vi "Test Broadcast Unfiltered Debug Log Not Filtered by Message.vi"(8 "error in (no error)":errorcluster, 11 "Test Case In":refnum<class "Debugger Test.lvclass">) -> (0 "error out":errorcluster, 3 "Test Case Out":refnum<class "Debugger Test.lvclass">)   [LabVIEW 2020, in "Debugger Test.lvclass"]
uses:
  Debugger Test.lvclass
  C:/Program Files (x86)/National Instruments/LabVIEW 2020/vi.lib/Astemes/LUnit/Test Case.lvclass
  source/Debugger/Debugger.lvclass
  C:/Users/anton/Documents/GitHub/triarc-debugger/source/Process/Debug Process.lvclass
  source/Debug Data/Raw Debug Data.ctl
  source/Debug Data/Debug Data.lvclass/Debug Data.ctl
  source/Process/Debug Process.lvclass/Debug Process.ctl
  <vilib>/Astemes/LUnit/Test Case.lvclass/Test Case.ctl
  <vilib>/Astemes/LUnit/LUnit Assertion Result.lvclass/LUnit Assertion Result.ctl
  <vilib>/Astemes/LUnit/LUnit Test Case Result.lvclass/LUnit Test Case Result.ctl
  <vilib>/Astemes/LUnit/LUnit Method Result.lvclass/LUnit Method Result.ctl
  01074fa8-ee8a-411d-bc8b-fc92c4f90959.vi
  source/Process/Public/Lifecycle/Get Lifecycle State.vi
  source/Process/Private/SubVIs/Wait for finish.vi
  source/Process/Protected/Messaging/Enqueue Message.vi
  source/Process/Private/SubVIs/Set Lifecycle State.vi
  <vilib>/Astemes/LUnit/Palette/Pass.vi
  <vilib>/Astemes/LUnit/Palette/Fail.vi
  <vilib>/Astemes/LUnit/Compare Variants.vi
  <vilib>/Astemes/LUnit/Describe Comparison.vi
  <vilib>/Astemes/LUnit/Set Assertion Type.vi
  <vilib>/Utility/error.llb/Clear Errors.vi
  <vilib>/Astemes/LUnit/Add test result.vi
  <vilib>/Astemes/LUnit/LUnit Write Passed.vi
  <vilib>/Astemes/LUnit/LUnit Write Message.vi
  <vilib>/Astemes/LUnit/LUnit Write Description.vi
  <vilib>/Astemes/LUnit/Variant to string.vi
  <vilib>/Astemes/LUnit/LUnit Write Assertion Type.vi
  <vilib>/Astemes/LUnit/LUnit Record Assertion Result.vi
  <vilib>/Astemes/LUnit/LUnit Aggregate Assertion Results.vi
  <vilib>/Astemes/LUnit/Assertion Result/LUnit Read Status.vi
  <vilib>/Astemes/LUnit/LUnit Read Message.vi
  <vilib>/Astemes/LUnit/LUnit Read Description.vi
  <vilib>/Astemes/LUnit/Method Result/LUnit Merge Status.vi
  <vilib>/Astemes/LUnit/LUnit Concatenate result strings.vi
  <vilib>/Utility/error.llb/Error Cluster From Error Code.vi
  <vilib>/Utility/Data Type/Get Type Information.vi
  <vilib>/Utility/LVClass/Get LV Class Name.vi
  <vilib>/Astemes/LUnit/LUnit Assertion Result.lvclass
  source/Process/Debug Process.lvclass
  source/Debug Data/Debug Data.lvclass
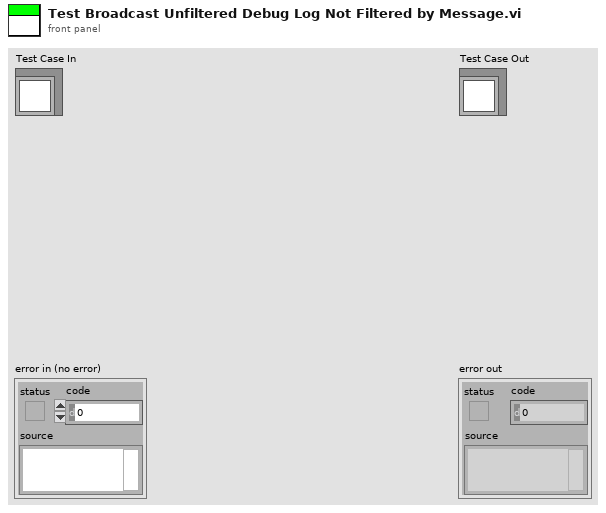
[diagram p1: front panel]
types:
  T1 = typedef "Debug Data.lvclass/Raw Debug Data.ctl" = cluster{"Action":string, "Call Chain":string, "Process":string, "Message":string, "Message Data":variant, "Time":dbl}
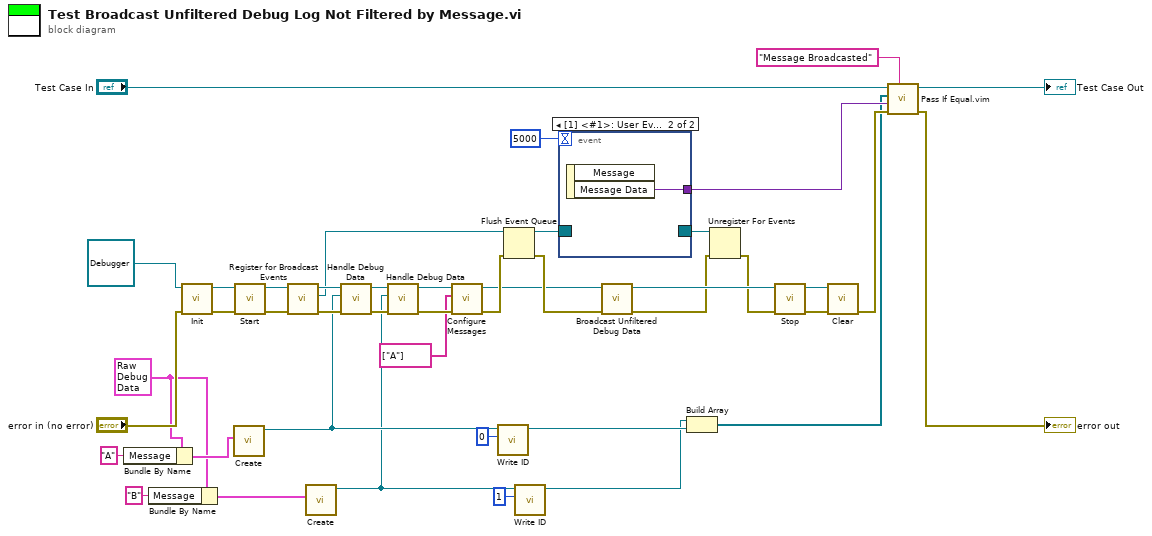
[diagram p0: block diagram]
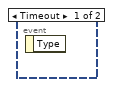
[diagram p2: hidden frame]
diagram:
  w12 = T1 {"Action"="", "Call Chain"="", "Process"="", "Message"="", "Message Data"=variant, "Time"=0.0} ("Debug Data Cluster")
  n1 = Bundle By Name(cluster=w12, "Message"="A" ("Process")) -> (w19:T1)
  n2 = Bundle By Name(cluster=w12, "Message"="B" ("Process")) -> (w13:T1)
  n3 = call-dynamic "Init.vi"("error in (no error)"="error in (no error)", "Process In"=refnum<class "Debugger.lvclass"> refnum ("Debug Data Event In 2")) -> ("error out"=w39:errorcluster, "Process Out"=w40:refnum<class "Debugger.lvclass">)  [unwired: 8 in]
  n4 = call "Create.vi"("Debug Data Cluster"=w19) -> ("Debug Data out"=w25:refnum<class "Debug Data.lvclass">)  [unwired: 9 in, 1 out]
  n5 = call "Start.vi"("error in (no error)"=w39, "Process In"=w40) -> ("error out"=w37:errorcluster, "Process Out"=w38:refnum<class "Debugger.lvclass">)  [unwired: 7 in, 1 out]
  n6 = call "Register for Broadcast Events.vi"("error in (no error)"=w37, "Process In"=w38) -> ("error out"=w36:errorcluster, "Event Registration Refnum Out"=w21:refnum<event-registration>, "Process Out"=w32:refnum<class "Debugger.lvclass">)  [unwired: 7 in]
  n7 = call "Create.vi"("Debug Data Cluster"=w13) -> ("Debug Data out"=w7:refnum<class "Debug Data.lvclass">)  [unwired: 9 in, 1 out]
  n8 = call-dynamic "Handle Debug Data.vi"("error in (no error)"=w36, "Debug Data.lvclass"=w25, "Debug Data Event In"=w32) -> ("error out"=w16:errorcluster, "Debug Data Event Out"=w17:refnum<class "Debugger.lvclass">)  [unwired: 7 in]
  n9 = call-dynamic "Handle Debug Data.vi"("error in (no error)"=w16, "Debug Data.lvclass"=w7, "Debug Data Event In"=w17) -> ("error out"=w15:errorcluster, "Debug Data Event Out"=w10:refnum<class "Debugger.lvclass">)  [unwired: 7 in]
  n10 = call "Configure Messages.vi"("error in (no error)"=w15, "Messages"=string[] ["A"], "Debugger In"=w10) -> ("error out"=w11:errorcluster, "Debugger Out"=w9:refnum<class "Debugger.lvclass">)  [unwired: 7 in]
  n11 = call "Write ID.vi"("ID"=u32 0, "Debug Data in"=w25) -> ("Debug Data out"=w4:refnum<class "Debug Data.lvclass">)  [unwired: 8 in, 1 out]
  n12 = Flush Event Queue(0:w21, 3:w11) -> (8:w20:refnum<event-registration>, 11:w22:errorcluster)  [unwired: 4 in, 1 out]
  n13 = call "Write ID.vi"("ID"=u32 1, "Debug Data in"=w7) -> ("Debug Data out"=w3:refnum<class "Debug Data.lvclass">)  [unwired: 8 in, 1 out]
  n14 = event shown="[1] <#1>: User Event" {
    selector: w20 -> [_ _]
    dyn-events: [_ _] -> w27
    timeout: 5000 -> [_ _]
    tunnel: [_ w44] -> w24
    event Timeout {
      n15 = event-data() -> ()  [unwired: 1 in, 1 out]
    }
    event User Event {
      n16 = event-data() -> ("Message Data"=w44:variant)  [unwired: 1 in, 1 out]
    }
  }
  n17 = call "Broadcast Unfiltered Debug Data.vi"("error in (no error)"=w22, "Debugger in"=w9) -> ("error out"=w6:errorcluster, "Debugger out"=w35:refnum<class "Debugger.lvclass">)  [unwired: 8 in]
  n18 = Build Array(w3, w4) -> (w23:refnum<class "Debug Data.lvclass">[])
  n19 = Unregister For Events(event registration refnum=w27, error in=w6) -> (error out=w5:errorcluster)
  n20 = call "Stop.vi"("error in (no error)"=w5, "Process In"=w35) -> ("error out"=w33:errorcluster, "Process Out"=w34:refnum<class "Debugger.lvclass">)  [unwired: 7 in, 1 out]
  n21 = call-dynamic "Clear.vi"("error in (no error)"=w33, "Process In"=w34) -> ("error out"=w29:errorcluster)  [unwired: 9 in]
  n22 = call "Pass If Equal.vim"("Description"="Message Broadcasted", "error in (no error)"=w29, "Actual"=w24, "Expected"=w23, "LUnit Test Case In"="Test Case In") -> ("error out"=→"error out":errorcluster, "LUnit Test Case Out"=→"Test Case Out":refnum<class "Debugger Test.lvclass">)  [unwired: 5 in]
